vi "Configure TLS.vi"(8 "error in (no error)":errorcluster, 9 "Use OS Certificates":bool, 10 "Cert Chains":T1(array[cluster]), 11 "Websocket Client in":refnum<class "Websocket Client.lvclass">) -> (0 "error out":errorcluster, 3 "Websocket Client out":refnum<class "Websocket Client.lvclass">)   [LabVIEW 2020, in "Stream-Websocket.lvlib" / "Websocket Client.lvclass"]
uses:
  Websocket Client.lvclass
  Websocket Client.lvclass/Websocket Client.ctl
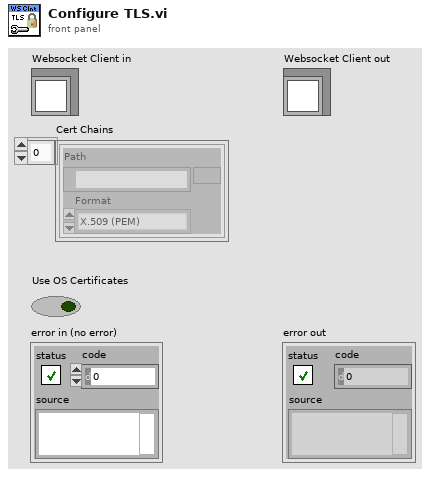
[diagram p1: front panel]
types:
  T1 = cluster{"Path":path, "Format":enum32{"X.509 (PEM)"}}[]
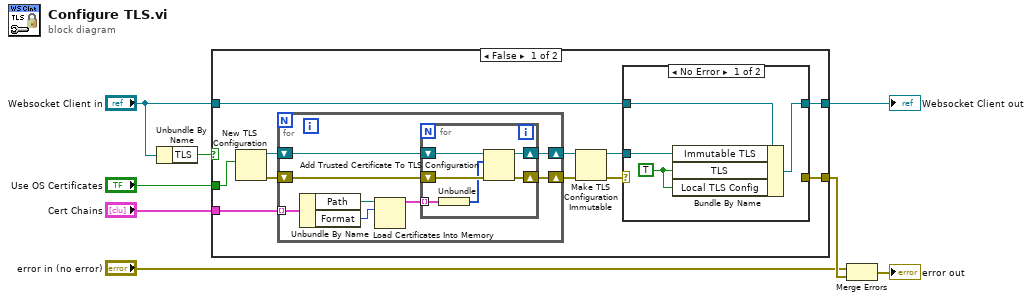
[diagram p0: block diagram]
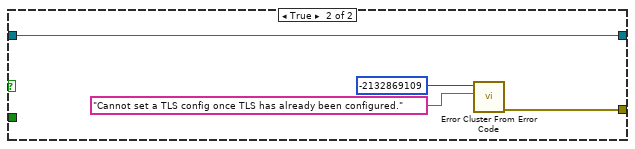
[diagram p3: hidden frame]
diagram:
  n1 = Unbundle By Name("Websocket Client in") -> ("TLS"=w1:bool)
  n2 = case shown="False" w1 {
    tunnel: "Websocket Client in" -> [w13 w43]
    tunnel: [w11 w43] -> w4
    tunnel: [w14 w40] -> w8
    tunnel: "Use OS Certificates" -> [w10 _]
    tunnel: "Cert Chains" -> [w9 _]
    frame False {
      n3 = New TLS Configuration(10:w10) -> (0:w19:errorcluster, 3:w18:refnum<k36>)  [unwired: 1 in]
      n4 = for {
        shift-right: [w27] -> w17
        shift-left: w19 -> [w28]
        shift-right: [w29] -> w16
        shift-left: w18 -> [w30]
        tunnel: w9 -> [w33] mode=indexing
        n5 = Unbundle By Name(w33) -> ("Path"=w32:path, "Format"=w31:enum32{"X.509 (PEM)"})
        n6 = Load Certificates Into Memory(10:w31, 11:w32) -> (3:w26:cluster{"certificate":u8[]}[])  [unwired: 1 in, 1 out]
        n7 = for {
          shift-right: [w38] -> w29
          shift-left: w30 -> [w39]
          shift-right: [w36] -> w27
          shift-left: w28 -> [w37]
          tunnel: w26 -> [w35] mode=indexing
          n8 = Unbundle(w35) -> ("certificate"=w34:u8[])
          n9 = Add Trusted Certificate To TLS Configuration(8:w37, 10:w34, 11:w39) -> (0:w36:errorcluster, 3:w38:refnum<k36>)
        }
      }
      n10 = Make TLS Configuration Immutable(8:w17, 11:w16) -> (0:w15:errorcluster, 3:w12:refnum<k36>)
      n11 = case shown="No Error" w15 {
        selector: w15 -> [_ w25]
        tunnel: [_ w25] -> w14
        tunnel: w13 -> [w23 w24]
        tunnel: w12 -> [w22 _]
        tunnel: [w21 w24] -> w11
        frame No Error {
          w20 = TRUE ("TLS")
          n12 = Bundle By Name(cluster=w23, "Immutable TLS"=w22, "TLS"=w20, "Local TLS Config"=w20) -> (w21:refnum<class "Websocket Client.lvclass">)
        }
        frame Error {
        }
      }
    }
    frame True {
      n13 = call <vilib>:"Error Cluster From Error Code.vi"("error message (\"\")"="Cannot set a TLS config once TLS has already been configured." ("error message (\"\")"), "error code (0)"=-2132869109) -> ("error out"=w40:errorcluster)  [unwired: 7 in]
    }
  }
  "Websocket Client out" <- w4
  n14 = Merge Errors("error in (no error)", w8) -> (→"error out":errorcluster)
